vi "FTP自动升级更新main.vi"() -> ()   [LabVIEW 2016, in "自动更新.lvlib"]
uses:
  <vilib>/FTP/NI_FTP.lvlib
panel:
  out "有新版本":bool
  out "最新版本获取进度":u8(slide) scale=0.0..100.0
  # "版本获取中，请稍后！"
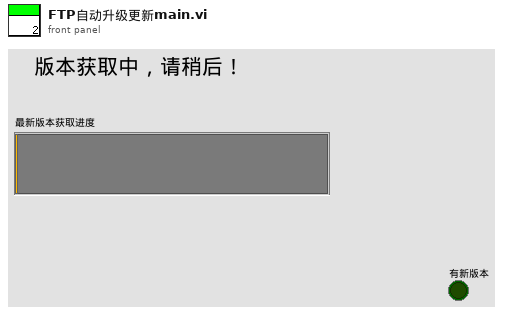
[diagram p1: front panel]
types:
  T1 = enum16{"get version information", "get success", "contact", "over"}
  T2 = cluster{"网络灯":bool, "接收中":bool, "已接收百分比":u8, "接收成功次数":dbl, "当前步骤":enum16{"init", "receivehead", "receivecontent", "receivesuccess", "over"}, "文件名":string, "error out":errorcluster}
  T3 = enum16{"open", "replace", "create", "open or create", "replace or create", "replace or create with confirmation"}
  T4 = cluster{"主机":string, "用户":string, "密码":string, "远程路径":string, "下载文件名":string, "软件版本":string}
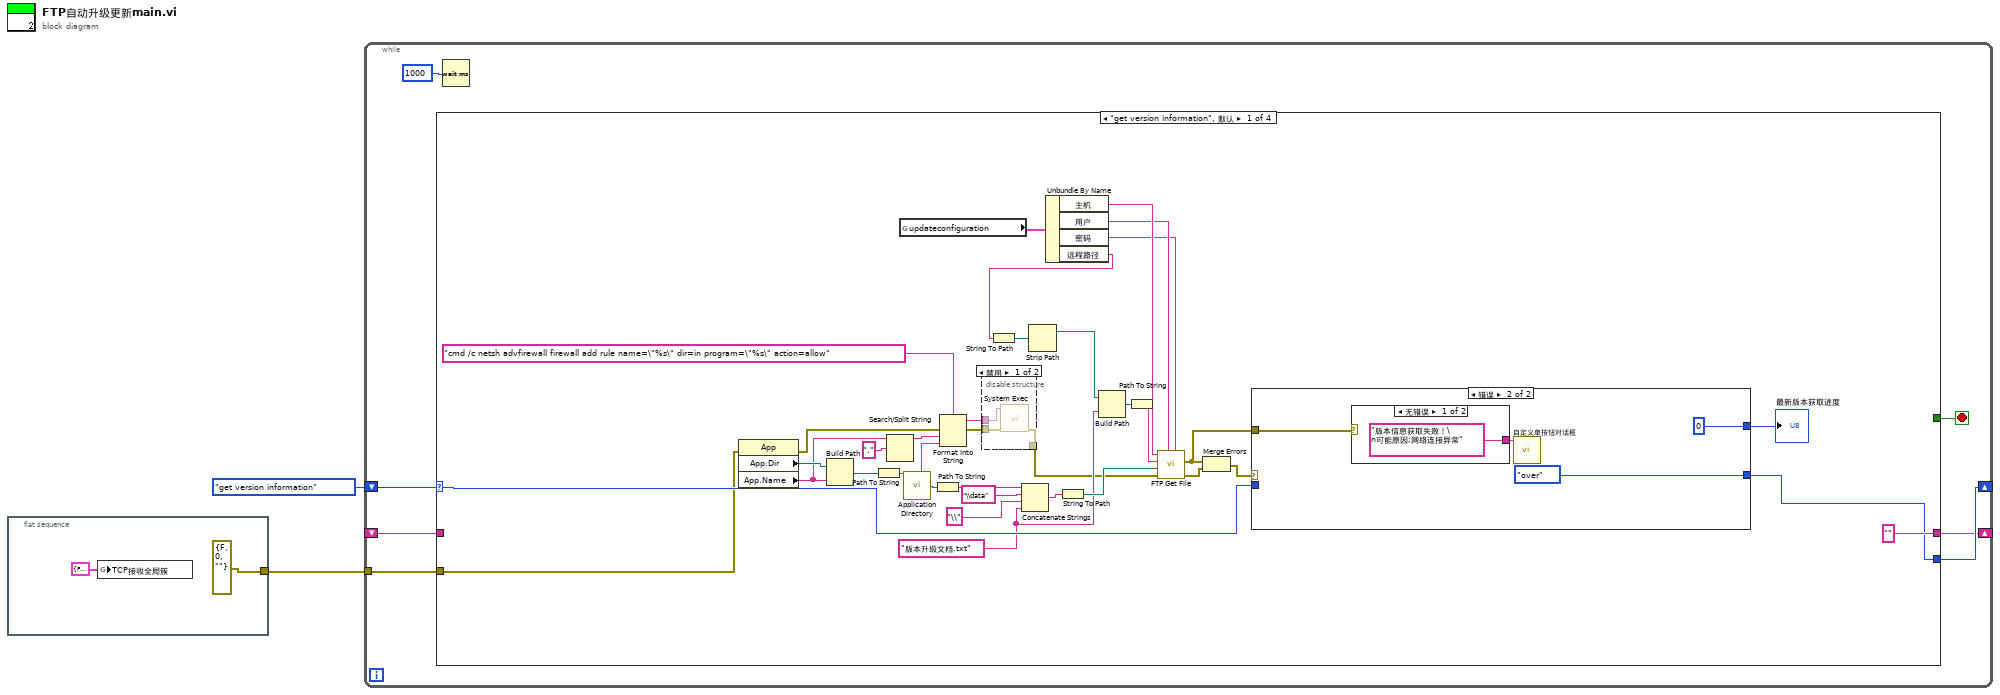
[diagram p0: block diagram]
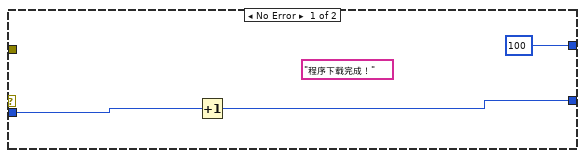
[diagram p3: hidden frame]
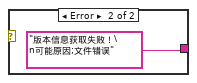
[diagram p4: hidden frame]
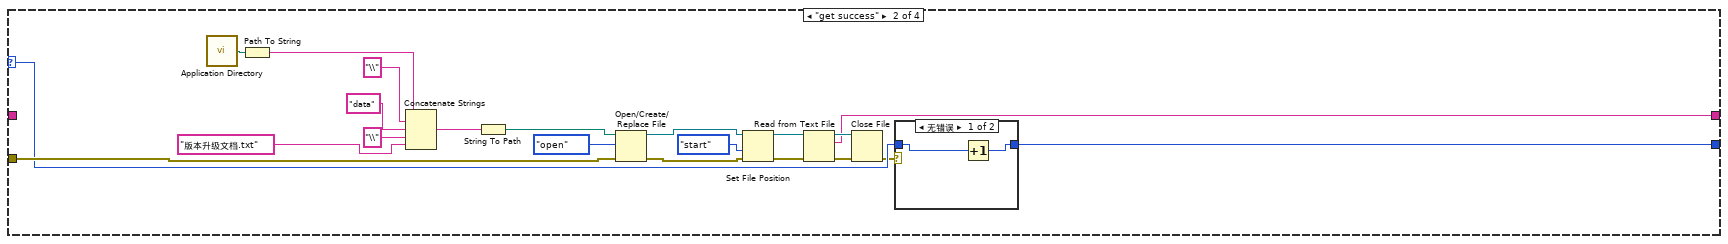
[diagram p5: hidden frame]
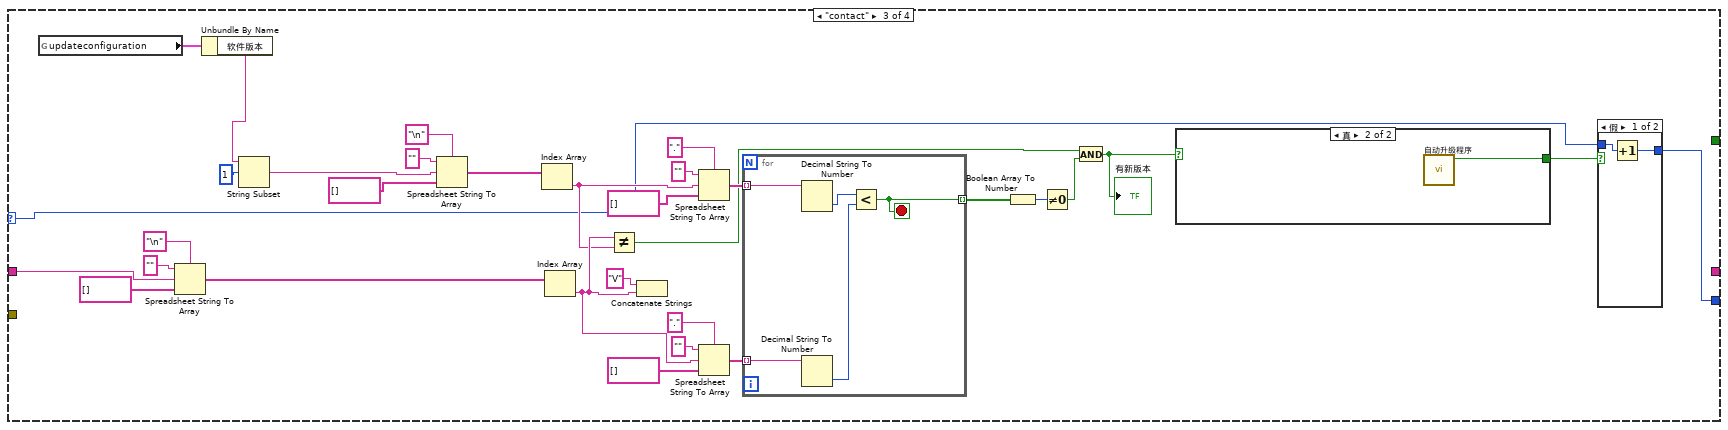
[diagram p7: hidden frame]
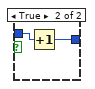
[diagram p8: hidden frame]
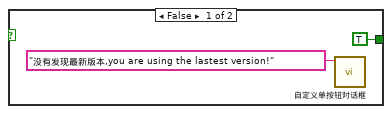
[diagram p9: hidden frame]
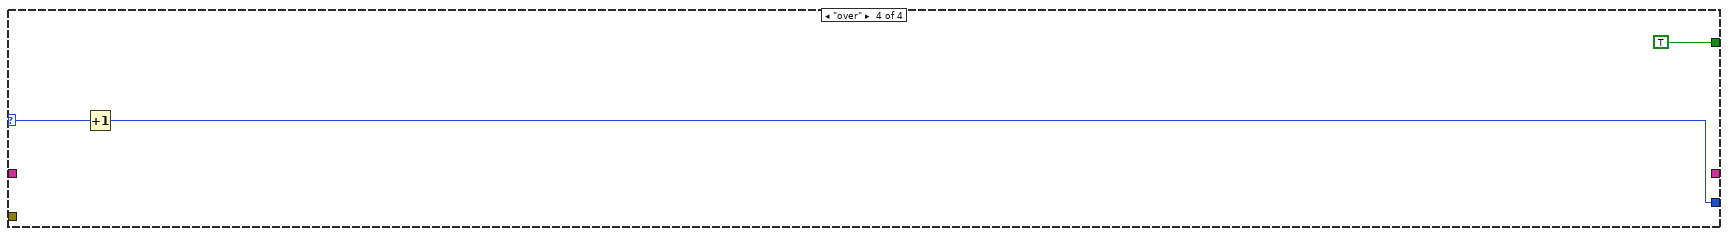
[diagram p10: hidden frame]
diagram:
  n1 = flat-sequence {
    tunnel: [errorcluster {"status"=FALSE, "code"=0, "source"=""} ("错误常量")] -> w1
    frame #0 {
      n2 = global write "全局变量1.vi" "TCP接收全局簇"(T2 {"网络灯"=FALSE, "接收中"=FALSE, "已接收百分比"=0, "接收成功次数"=0.0, "当前步骤"=enum."init", "文件名"="", "error out"={"status"=FALSE, "code"=0, "source"=""}} ("TCP接收全局簇")) -> ()
    }
  }
  n3 = while {
    shift-right: [w9] -> _
    shift-left: T1."get version information" -> [w10]
    tunnel: w1 -> [w8]
    shift-right: [w7] -> _
    shift-left: _ -> [w6]
    stop <- w5 stop-if-true
    n4 = case shown="\"get version information\", 默认" w10 {
      selector: w10 -> [w36 w66 w86 w128]
      tunnel: [w35 w65 w85 w127] -> w9
      tunnel: w8 -> [w12 w67 _ _]
      tunnel: ["" w59 _ _] -> w7
      tunnel: w6 -> [_ _ w89 _]
      tunnel: [_ _ _ TRUE] -> w5
      frame "get version information", Default {
        w26 = "版本升级文档.txt"
        n5 = property class="App"(error in=w12) -> (error out=w17:errorcluster, "App.Dir"=w23:path, "App.Name"=w19:string)  [unwired: 1 in, 1 out]
        n6 = Build Path(base path=w23, name or relative path=w19) -> (appended path=w22:path)
        n7 = Path To String(path=w22) -> (string=w21:string)
        n8 = Search/Split String(string=w19, search string/char (-)="." ("搜索字符串/字符(-)")) -> (substring before match=w18:string)  [unwired: 1 in, 2 out]
        n9 = global read "update全局.vi" "updateconfiguration"() -> (w34:T4)
        n10 = call <vilib>:"Application Directory.vi"() -> ("Application Directory"=w43:path)
        n11 = Path To String(path=w43) -> (string=w45:string)
        n12 = Format Into String(format string="cmd /c netsh advfirewall firewall add rule name=\"%s\" dir=in program=\"%s\" action=allow" ("command line"), error in=w17, w18, w21) -> (resulting string=w14:string, error out=w16:errorcluster)  [unwired: 1 in]
        n13 = disable-structure shown="禁用" {
          disable-tunnel: w16 -> [w49 _]
          disable-tunnel: w14 -> [w48 _]
          disable-tunnel: [w47 _] -> w13
          frame Disabled {
            n14 = call <vilib>:"System Exec.vi"("error in (no error)"=w49, "command line"=w48) -> ("error out"=w47:errorcluster)  [unwired: 6 in, 3 out]
          }
          frame Enabled {
          }
        }
        n15 = Concatenate Strings(w45, "\\data" ("字符串"), "\\" ("字符串"), w26) -> (w42:string)
        n16 = Unbundle By Name(w34) -> ("主机"=w33:string, "用户"=w32:string, "密码"=w31:string, "远程路径"=w27:string)
        n17 = String To Path(string=w27) -> (path=w29:path)
        n18 = Strip Path(path=w29) -> (stripped path=w28:path)  [unwired: 1 out]
        n19 = String To Path(string=w42) -> (path=w41:path)
        n20 = Build Path(base path=w28, name or relative path=w26) -> (appended path=w25:path)
        n21 = Path To String(path=w25) -> (string=w24:string)
        n22 = call <vilib>:"FTP Get File.vi"("password"=w31, "user"=w32, "error in (no error)"=w13, "local path"=w41, "remote path"=w24, "host"=w33) -> ("error out"=w40:errorcluster, "file error"=w38:errorcluster)  [unwired: 4 in]
        n23 = Merge Errors(w38, w40) -> (w39:errorcluster)
        n24 = case shown="错误" w39 {
          tunnel: w38 -> [_ w55]
          tunnel: [u8 100 ("y") u8 0 ("y")] -> w37
          tunnel: [w51 T1."over"] -> w35
          tunnel: w36 -> [w50 _]
          frame No Error {
            (unwired) "程序下载完成！"
            n25 = Increment(x=w50) -> (x+1=w51:T1)
          }
          frame Error {
            n26 = case shown="无错误" w55 {
              tunnel: ["版本信息获取失败！\n可能原因;网络连接异常" "版本信息获取失败！\n可能原因;文件错误"] -> w56
              frame No Error {
              }
              frame Error {
              }
            }
            n27 = call "自定义单按钮对话框.vi"("消息"=w56) -> ()  [unwired: 11 in]
          }
        }
        "最新版本获取进度" <- w37
      }
      frame "get success" {
        n28 = call <vilib>:"Application Directory.vi"() -> ("Application Directory"=w72:path)
        n29 = Path To String(path=w72) -> (string=w75:string)
        n30 = Concatenate Strings(w75, "\\" ("字符串"), "data" ("字符串"), "\\" ("字符串"), "版本升级文档.txt" ("字符串")) -> (w69:string)
        n31 = String To Path(string=w69) -> (path=w68:path)
        n32 = Open/Create/Replace File(file path (use dialog)=w68, error in=w67, operation (0:open)=T3."open" ("操作(0:open)")) -> (refnum out=w78:refnum<file>, error out=w77:errorcluster)  [unwired: 3 in, 1 out]
        n33 = Set File Position(refnum=w78, from (0:start)=enum16{"start", "end", "current"}."start" ("自（0:起始）"), error in=w77) -> (refnum out=w63:refnum<file>, error out=w62:errorcluster)  [unwired: 1 in]
        n34 = Read from Text File(file (use dialog)=w63, error in=w62) -> (refnum out=w64:refnum<file>, text=w59:string, error out=w61:errorcluster)  [unwired: 2 in, 1 out]
        n35 = Close File(refnum=w64, error in=w61) -> (error out=w60:errorcluster)  [unwired: 1 out]
        n36 = case shown="无错误" w60 {
          tunnel: w66 -> [w81 w82]
          tunnel: [w80 w82] -> w65
          frame No Error {
            n37 = Increment(x=w81) -> (x+1=w80:T1)
          }
          frame Error {
          }
        }
      }
      frame "contact" {
        n38 = global read "update全局.vi" "updateconfiguration"() -> (w84:T4)
        n39 = Spreadsheet String To Array(delimiter (Tab)="\n" ("分隔符(Tab)"), format string="" ("格式字符串"), spreadsheet string=w89, array type (2D Dbl)=string[] []) -> (array=w110:string[])
        n40 = Unbundle By Name(w84) -> ("软件版本"=w83:string)
        n41 = String Subset(string=w83, offset (0)=1 ("偏移量(0)")) -> (substring=w102:string)  [unwired: 1 in]
        n42 = Spreadsheet String To Array(delimiter (Tab)="\n" ("分隔符(Tab)"), format string="" ("格式字符串"), spreadsheet string=w102, array type (2D Dbl)=string[] []) -> (array=w101:string[])
        n43 = Index Array(array=w101) -> (element=w92:string)  [unwired: 1 in]
        n44 = Index Array(array=w110) -> (element=w93:string)  [unwired: 1 in]
        n45 = Not Equal?(x=w93, y=w92) -> (x != y?=w90:bool)
        n46 = Concatenate Strings("V" ("字符串"), w93) -> ()  [unwired: 1 out]
        n47 = Spreadsheet String To Array(delimiter (Tab)="." ("分隔符(Tab)"), format string="" ("格式字符串"), spreadsheet string=w92, array type (2D Dbl)=string[] []) -> (array=w96:string[])
        n48 = Spreadsheet String To Array(delimiter (Tab)="." ("分隔符(Tab)"), format string="" ("格式字符串"), spreadsheet string=w93, array type (2D Dbl)=string[] []) -> (array=w97:string[])
        n49 = for {
          tunnel: w97 -> [w124] mode=indexing
          tunnel: w96 -> [w126] mode=indexing
          tunnel: [w125] -> w95 mode=indexing
          stop <- w125 stop-if-true
          n50 = Decimal String To Number(string=w126) -> (number=w123:i32)  [unwired: 2 in, 1 out]
          n51 = Decimal String To Number(string=w124) -> (number=w122:i32)  [unwired: 2 in, 1 out]
          n52 = Less?(x=w123, y=w122) -> (x < y?=w125:bool)
        }
        n53 = Boolean Array To Number(Boolean array=w95) -> (number=w94:u32)
        n54 = Not Equal To 0?(x=w94) -> (x != 0?=w91:bool)
        n55 = And(x=w90, y=w91) -> (x .and. y?=w88:bool)
        "有新版本" <- w88
        n56 = case shown="真" w88 {
          tunnel: [TRUE ("确定") w121] -> w87
          frame False {
            n57 = call "自定义单按钮对话框.vi"("消息"="没有发现最新版本,you are using the lastest version!") -> ()  [unwired: 11 in]
          }
          frame True {
            n58 = call "自动升级程序.vi"() -> ("确定"=w121:bool)  [unwired: 10 in, 1 out]
          }
        }
        n59 = case shown="假" w87 {
          tunnel: w86 -> [w116 w118]
          tunnel: [w115 w117] -> w85
          frame False {
            n60 = Increment(x=w116) -> (x+1=w115:T1)
          }
          frame True {
            n61 = Increment(x=w118) -> (x+1=w117:T1)
          }
        }
      }
      frame "over" {
        n62 = Increment(x=w128) -> (x+1=w127:T1)
      }
    }
    n63 = Wait (ms)(milliseconds to wait=u32 1000 ("等待时间（毫秒）")) -> ()  [unwired: 1 out]
  }
